vi "Delete Edge.vi"(0 "FSM.Graph In":refnum<class "FSM.Graph.lvclass">) -> (4 "FSM.Graph Out":refnum<class "FSM.Graph.lvclass">, 8 "Deleted Edge":refnum<class "FSM.Edge.lvclass">)   [LabVIEW 2020, in "FSM.Graph.lvclass"]
uses:
  FSM.Graph.lvclass
  FSM.Edge/FSM.Edge.lvclass
  FSM.Graph.lvclass/FSM.Graph.ctl
  FSM.Edge/FSM.Edge.lvclass/FSM.Edge.ctl
  FSM.Edge/Read SourceName.vi
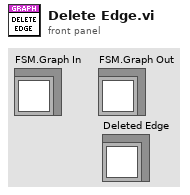
[diagram p1: front panel]
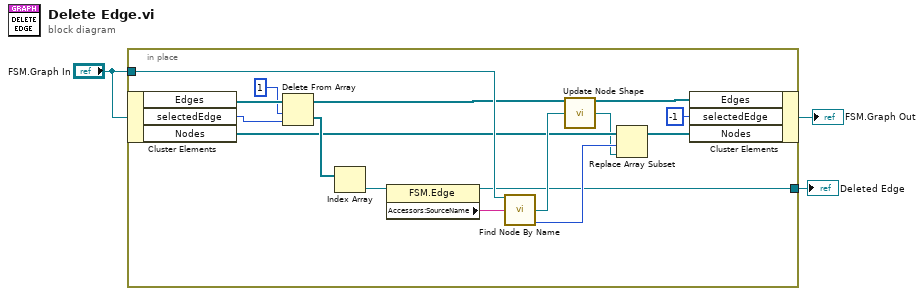
[diagram p0: block diagram]
diagram:
  n1 = in-place {
    in-place-border: "FSM.Graph In" -> [w11]
    in-place-border: [w4] -> w1
    n2 = in-place-cluster #1("FSM.Graph In") -> ("Edges"=w19:refnum<class "FSM.Edge.lvclass">[], "selectedEdge"=w18:i32, "Nodes"=w8:refnum<class "FSM.Node.lvclass">[])
    n3 = Delete From Array(array=w19, length=1, index=w18) -> (deleted portion=w12:refnum<class "FSM.Edge.lvclass">[], array with subset deleted=w10:refnum<class "FSM.Edge.lvclass">[])
    n4 = Index Array(array=w12) -> (element=w15:refnum<class "FSM.Edge.lvclass">)  [unwired: 1 in]
    n5 = property class="FSM.Edge"(reference=w15) -> (reference out=w4:refnum<class "FSM.Edge.lvclass">, "Accessors:SourceName"=w14:string)  [unwired: 1 in, 1 out]
    n6 = call "Find Node By Name.vi"("FSM.Graph"=w11, "Name"=w14) -> ("Node"=w13:refnum<class "FSM.Node.lvclass">, "index"=w6:i32)  [unwired: 12 in]
    n7 = call "Update Node Shape.vi"("Edges"=w10, "FSM.Node in"=w13) -> ("Edges Out"=w9:refnum<class "FSM.Edge.lvclass">[], "FSM.Node out"=w5:refnum<class "FSM.Node.lvclass">)  [unwired: 12 in]
    n8 = Replace Array Subset(array=w8, new element=w5, index=w6) -> (w7:refnum<class "FSM.Node.lvclass">[])
    n9 = in-place-cluster #1("Edges"=w9, "selectedEdge"=-1, "Nodes"=w7) -> (→"FSM.Graph Out":refnum<class "FSM.Graph.lvclass">)
  }
  "Deleted Edge" <- w1
